vi "RunOperation.vi"(10 "Inputs":string[](array[string]), 11 "UniquifyFullyQualifiedVIName in":refnum<class "UniquifyFullyQualifiedVIName.lvclass">) -> (1 "Output/Failure":string, 2 "CLI Process Return Code":i32, 3 "UniquifyFullyQualifiedVIName out":refnum<class "UniquifyFullyQualifiedVIName.lvclass">)   [LabVIEW 2015, in "UniquifyFullyQualifiedVIName.lvclass"]
uses:
  UniquifyFullyQualifiedVIName.lvclass
  UniquifyFullyQualifiedVIName.lvclass/UniquifyFullyQualifiedVIName.ctl
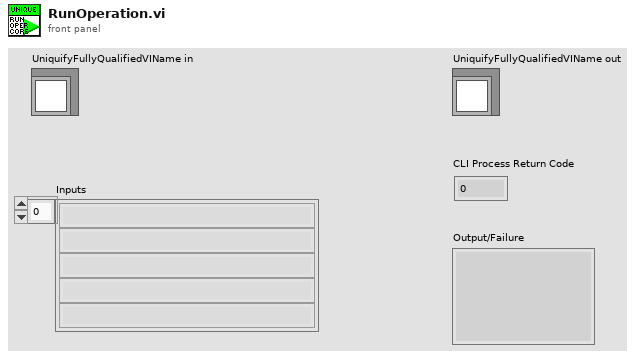
[diagram p1: front panel]
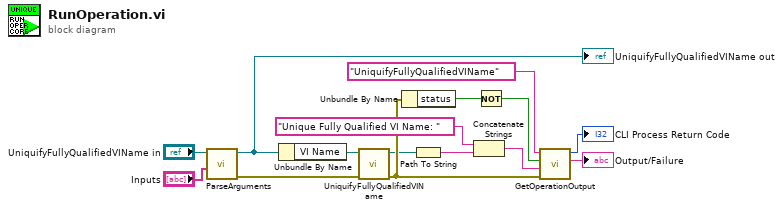
[diagram p0: block diagram]
diagram:
  n1 = call "ParseArguments.vi"("Inputs"="Inputs", "UniquifyFullyQualifiedVIName in"="UniquifyFullyQualifiedVIName in") -> ("error out"=w13:errorcluster, "UniquifyFullyQualifiedVIName out"=w12:refnum<class "UniquifyFullyQualifiedVIName.lvclass">)  [unwired: 8 in]
  "UniquifyFullyQualifiedVIName out" <- w12
  n2 = Unbundle By Name(w12) -> ("VI Name"=w11:path)
  n3 = call "UniquifyFullyQualifiedVIName.vi"("error in (no error)"=w13, "vi path"=w11) -> ("error out"=w8:errorcluster, "uniquified vi path"=w4:path)  [unwired: 8 in]
  n4 = Unbundle By Name(w8) -> ("status"=w10:bool)
  n5 = Path To String(path=w4) -> (string=w3:string)
  n6 = Concatenate Strings("Unique Fully Qualified VI Name: " ("string"), w3) -> (w1:string)
  n7 = Not(x=w10) -> (.not. x?=w9:bool)
  n8 = call <nishared>:"GetOperationOutput.vi"("error in (no error)"=w8, "Operation Output/Error In"=w1, "Operation succeeded?"=w9, "Operation Name"="UniquifyFullyQualifiedVIName") -> ("Operation Output/Error Out"=→"Output/Failure":string, "CLI Process Return Code"=→"CLI Process Return Code":i32)  [unwired: 6 in]
